vi "Sndbox algo.vi"() -> ()   [LabVIEW 2019]
uses:
  Modbus_class/CMD REG.ctl
  5f95f8ce-56eb-4e93-948d-6cc3724d9d28.vi
  f9ad96a4-e216-42df-aa27-456f2a66aeca.vi
panel:
  out "Array":string[](array[string])
  in  "CMD REG":T1
  out "t out":dbl
  in  "stop":bool
  out "Error":dbl=-0.0025653406548507007
  in  "I":dbl=0.5207744324250397
  in  "T1":dbl=10.0
  in  "K1":dbl=62.0
  in  "P sp":dbl=30.0
  out "Voltage":dbl(graph)
  in  "N":i32=1
  out "Pressure":cluster{"P pv":dbl, "P sp":dbl}(graph)
  out "dP":dbl
  in  "P pv":dbl
  out "R * U":dbl=35.930584668072186
  in  "U":dbl
  in  "K0":dbl=69.0
  in  "P0":dbl=6.0
  in  "T0":dbl=50.0
  in  "dt":dbl=0.1
  # "571,7"
  # "1141,5"
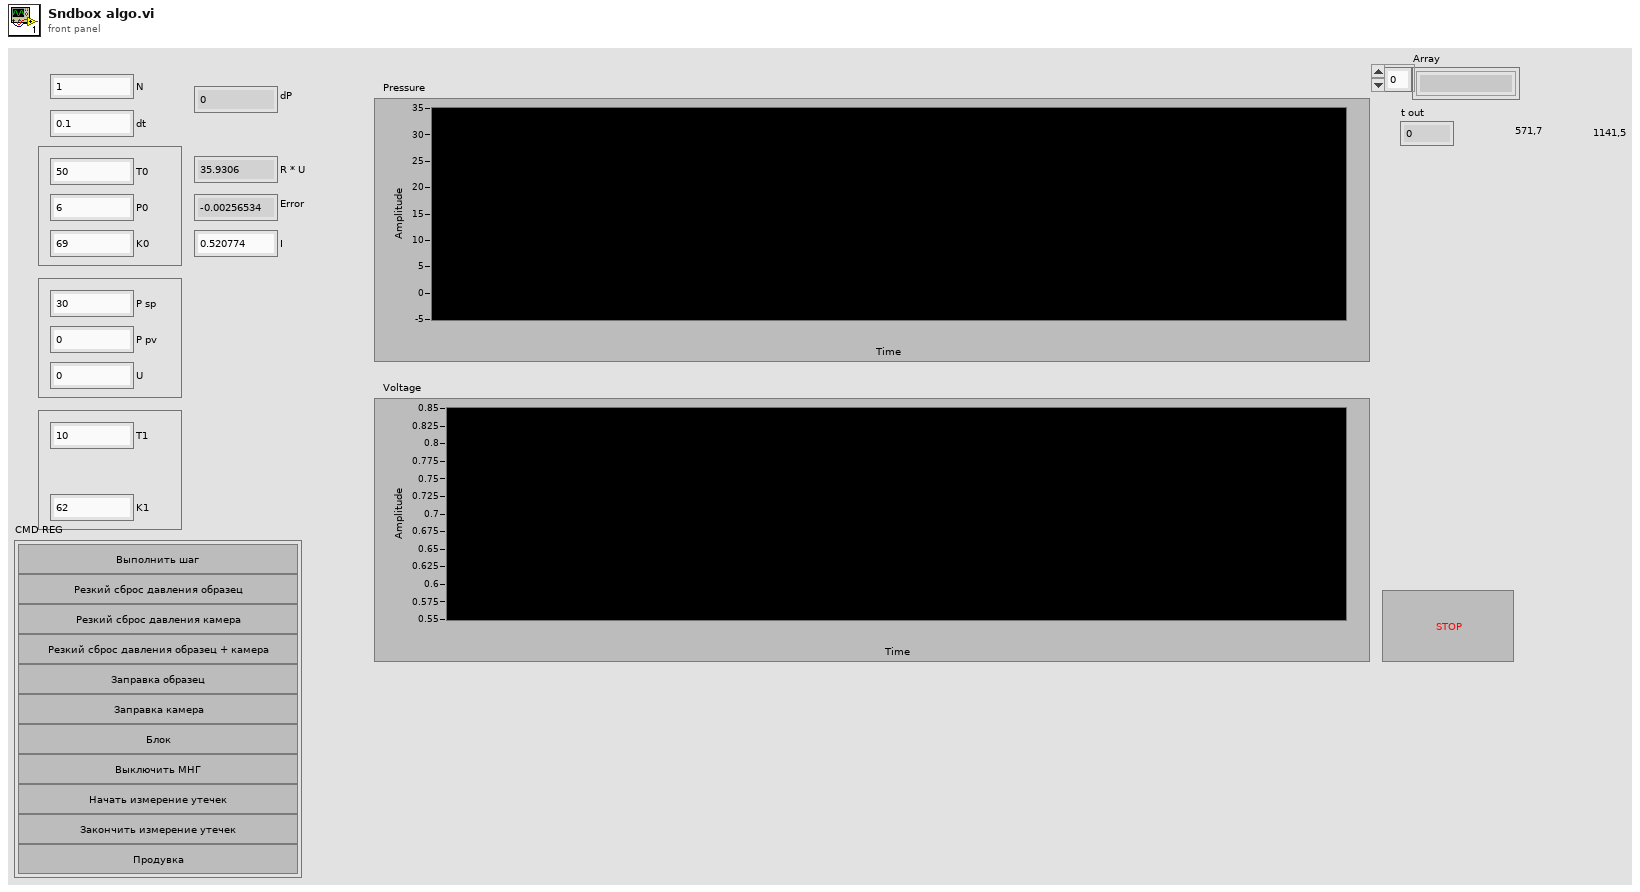
[diagram p1: front panel]
types:
  T1 = typedef "CMD REG.ctl" = cluster{"EXECUTE_SP":bool, "ALARM_PRESS_DOWN_DUT":bool, "ALARM_PRESS_DOWN_CHAMBER":bool, "ALARM_PRESS_DOWN_DUT_CHAMBER":bool, "FILING_DUT":bool, "FILING_CHAMBER":bool, "BLOCK":bool, "PUMP_STATION_OFF":bool, "Leak start":bool, "Leak stop":bool, "Drain":bool}
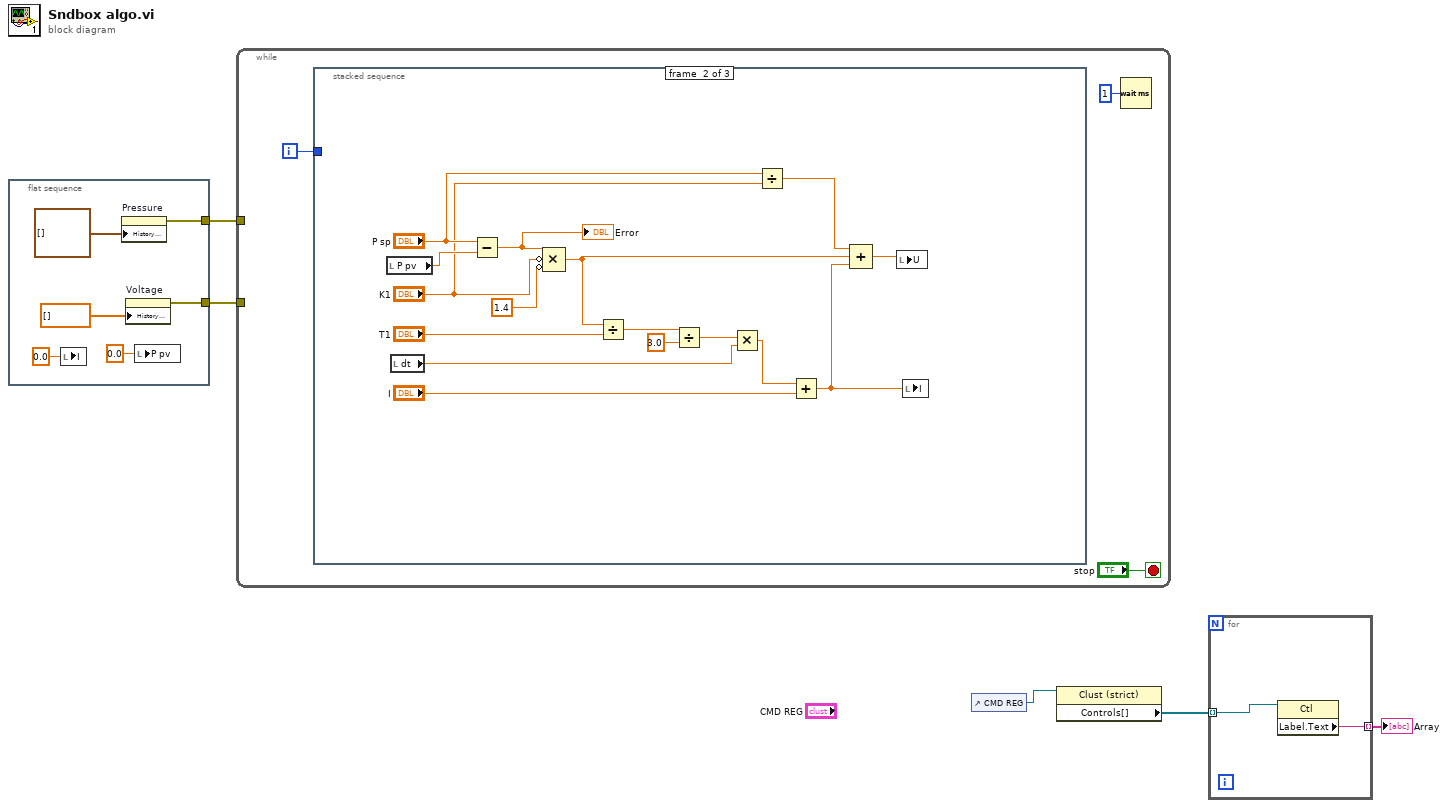
[diagram p0: block diagram]
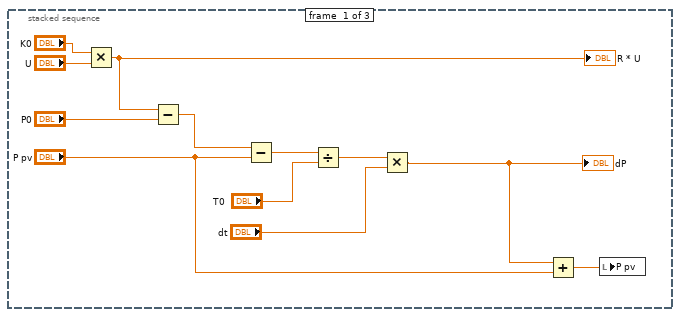
[diagram p2: hidden frame]
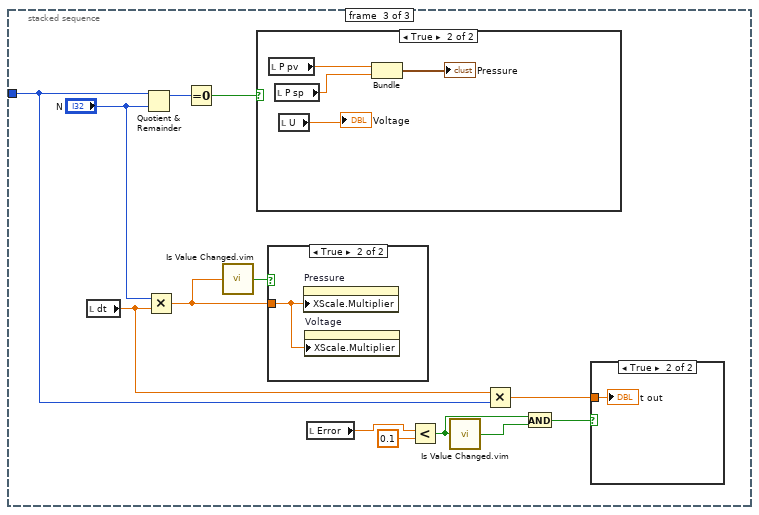
[diagram p3: hidden frame]
diagram:
  n1 = flat-sequence {
    tunnel: [w10] -> w5
    tunnel: [w8] -> w4
    frame #0 {
      n2 = local write "I"(0.0 ("I")) -> ()
      n3 = property on="Pressure" class="WFChart (strict)"("History Data"=cluster{"P pv":dbl, "P sp":dbl}[] []) -> (error out=w8:errorcluster)  [unwired: 2 in, 1 out]
      n4 = property on="Voltage" class="WFChart (strict)"("History Data"=dbl[] []) -> (error out=w10:errorcluster)  [unwired: 2 in, 1 out]
      n5 = local write "P pv"(0.0 ("P pv")) -> ()
    }
  }
  n6 = while {
    tunnel: w5 -> [_]
    tunnel: w4 -> [_]
    i -> [w13]
    stop <- "stop" stop-if-true
    n7 = stacked-sequence {
      tunnel: w13 -> [_ _ w44]
      frame #0 {
        n8 = Multiply(x="K0", y="U") -> (x*y=w24:dbl)
        "R * U" <- w24
        n9 = Subtract(x=w24, y="P0") -> (x-y=w22:dbl)
        n10 = Subtract(x=w22, y="P pv") -> (x-y=w21:dbl)
        n11 = Divide(x=w21, y="T0") -> (x/y=w19:dbl)
        n12 = Multiply(x=w19, y="dt") -> (x*y=w16:dbl)
        "dP" <- w16
        n13 = Add(x=w16, y="P pv") -> (x+y=w17:dbl)
        n14 = local write "P pv"(w17) -> ()
      }
      frame #1 {
        n15 = local read "P pv"() -> (w42:dbl)
        n16 = local read "dt"() -> (w31:dbl)
        n17 = Subtract(x="P sp", y=w42) -> (x-y=w32:dbl)
        "Error" <- w32
        n18 = Compound Arithmetic op=MULTIPLY(w32, invert "K1", invert 1.4 ("value")) -> (w34:dbl)
        n19 = Divide(x=w34, y="T1") -> (x/y=w40:dbl)
        n20 = Divide(x=w40, y=3.0) -> (x/y=w38:dbl)
        n21 = Multiply(x=w38, y=w31) -> (x*y=w37:dbl)
        n22 = Divide(x="P sp", y="K1") -> (x/y=w28:dbl)
        n23 = Add(x=w37, y="I") -> (x+y=w35:dbl)
        n24 = Compound Arithmetic op=ADD(w28, w34, w35) -> (w33:dbl)
        n25 = local write "U"(w33) -> ()
        n26 = local write "I"(w35) -> ()
      }
      frame #2 {
        n27 = local read "dt"() -> (w45:dbl)
        n28 = Quotient & Remainder(x=w44, y="N") -> (x-y*floor(x/y)=w52:i32)  [unwired: 1 out]
        n29 = Multiply(x="N", y=w45) -> (x*y=w54:dbl)
        n30 = Equal To 0?(x=w52) -> (x = 0?=w51:bool)
        n31 = call "Is Value Changed.vim"("value"=w54) -> ("changed or first call?"=w55:bool)
        n32 = case shown="True" w51 {
          frame False {
          }
          frame True {
            n33 = local read "P pv"() -> (w60:dbl)
            n34 = local read "P sp"() -> (w57:dbl)
            n35 = local read "U"() -> (→"Voltage":dbl)
            n36 = Bundle("P pv"=w60, "P sp"=w57) -> (→"Pressure":cluster{"P pv":dbl, "P sp":dbl})  [unwired: 1 in]
          }
        }
        n37 = case shown="True" w55 {
          tunnel: w54 -> [_ w61]
          frame False {
          }
          frame True {
            n38 = property on="Pressure" class="WFChart (strict)"("XScale.Multiplier"=w61) -> ()  [unwired: 2 in, 2 out]
            n39 = property on="Voltage" class="WFChart (strict)"("XScale.Multiplier"=w61) -> ()  [unwired: 2 in, 2 out]
          }
        }
        n40 = local read "Error"() -> (w43:dbl)
        n41 = Less?(x=w43, y=0.1) -> (x < y?=w49:bool)
        n42 = call "Is Value Changed.vim"("value"=w49) -> ("changed or first call?"=w50:bool)
        n43 = Multiply(x=w45, y=w44) -> (x*y=w47:dbl)
        n44 = And(x=w49, y=w50) -> (x .and. y?=w48:bool)
        n45 = case shown="True" w48 {
          tunnel: w47 -> [_ w56]
          frame False {
          }
          frame True {
            "t out" <- w56
          }
        }
      }
    }
    n46 = Wait (ms)(milliseconds to wait=u32 1) -> ()  [unwired: 1 out]
  }
  n47 = control-ref of="CMD REG"() -> (w3:refnum<vi>)
  n48 = property class="Clust (strict)"(reference=w3) -> ("Controls[]"=w2:refnum<vi>[])  [unwired: 1 in, 2 out]
  n49 = for {
    tunnel: w2 -> [w63] mode=indexing
    tunnel: [w62] -> w1 mode=indexing
    n50 = property class="Ctl"(reference=w63) -> ("Label.Text"=w62:string)  [unwired: 1 in, 2 out]
  }
  "Array" <- w1
